vi "set_mirrors_from_EoF.vi"(1 "offset Y":dbl, 3 "offset X":dbl, 4 "Line_start":i32, 5 "Range":dbl=10.0, 6 "Pixels":i32=256, 7 "dwell":dbl=1.0) -> (0 "X and Y":waveform(dbl)[](array[waveform]), 2 "appended array":dbl[][](array[numeric]))   [LabVIEW 2016]
panel:
  out "start frame Y Volts 2":dbl
  out "Waveform Graph 2":dbl[](graph)
  out "start frame Y Volts":dbl
  out "Waveform Graph":waveform(dbl)[](graph)
  out "border of frame X Volts":dbl
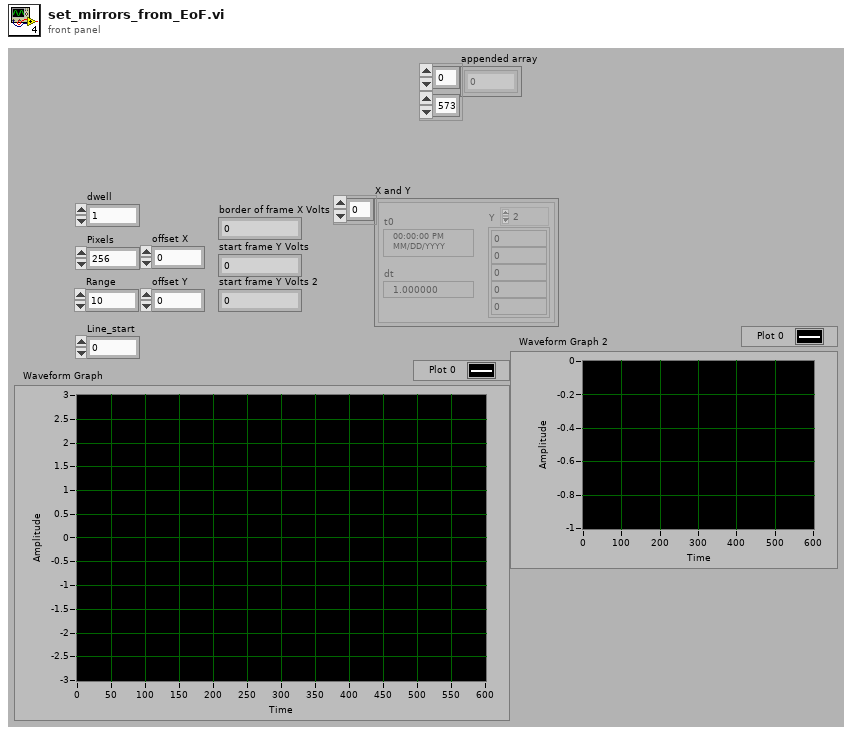
[diagram p1: front panel]
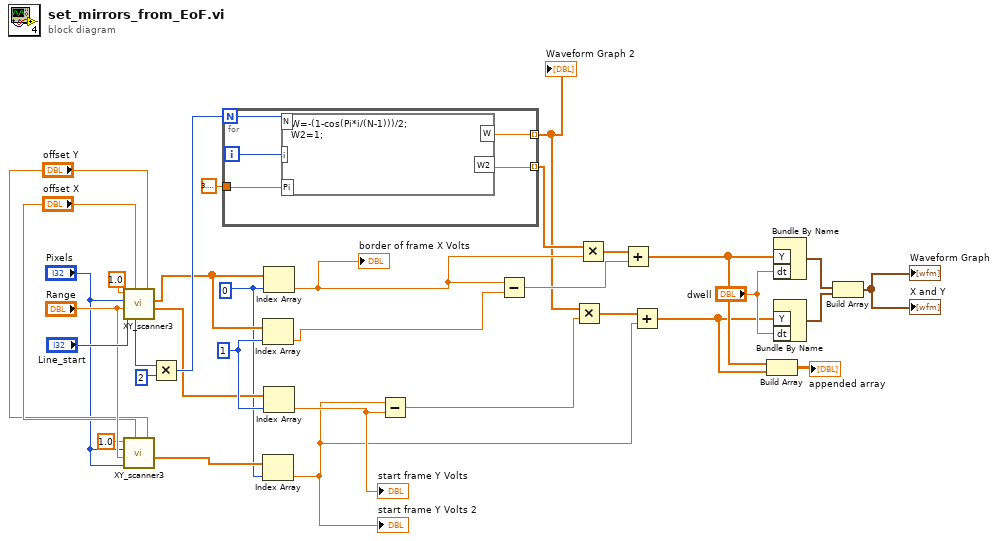
[diagram p0: block diagram]
diagram:
  w1 = 0 ("index")
  w3 = 1 ("index")
  n1 = call "XY_scanner3.vi"("offset Y"="offset Y", "offset X"="offset X", "Line_start"="Line_start", "Range"="Range", "Pixels"="Pixels", "dwell"=1.0) -> ("Array Y"=w2:dbl[], "Array X"=w4:dbl[], "scanPix"=w15:i32)  [unwired: 1 out]
  n2 = call "XY_scanner3.vi"("offset Y"="offset Y", "offset X"="offset X", "Line_start"="Pixels", "Range"="Range", "Pixels"="Pixels", "dwell"=1.0) -> ("Array Y"=w14:dbl[])  [unwired: 3 out]
  n3 = Multiply(x=w15, y=2) -> (x*y=w20:i32)
  n4 = for {
    N: w20 -> [w37]
    tunnel: 3.141592653589793 -> [w36]
    tunnel: [w35] -> w7 mode=indexing
    tunnel: [w34] -> w25 mode=indexing
    i -> [w38]
    n5 = formula code="W=-(1-cos(Pi*i/(N-1)))/2;\nW2=1;"("N"=w37, "i"=w38, "Pi"=w36) -> ("W"=w35:dbl, "W2"=w34:dbl)
  }
  "Waveform Graph 2" <- w7
  n6 = Index Array(array=w4, index=w3) -> (element=w12:dbl)
  n7 = Index Array(array=w14, index=w1) -> (element=w5:dbl)
  "start frame Y Volts 2" <- w5
  n8 = Index Array(array=w4, index=w1) -> (element=w11:dbl)
  "border of frame X Volts" <- w11
  n9 = Index Array(array=w2, index=w3) -> (element=w6:dbl)
  "start frame Y Volts" <- w6
  n10 = Subtract(x=w5, y=w6) -> (x-y=w8:dbl)
  n11 = Subtract(x=w11, y=w12) -> (x-y=w24:dbl)
  n12 = Multiply(x=w7, y=w8) -> (x*y=w10:dbl[])
  n13 = Multiply(x=w25, y=w11) -> (x*y=w23:dbl[])
  n14 = Add(x=w23, y=w24) -> (x+y=w22:dbl[])
  n15 = Add(x=w10, y=w5) -> (x+y=w9:dbl[])
  n16 = Build Array(w22, w9) -> (→"appended array":dbl[][])
  n17 = Bundle By Name("Y"=w22, "dt"="dwell") -> (w31:waveform(dbl))  [unwired: 1 in]
  n18 = Bundle By Name("Y"=w9, "dt"="dwell") -> (w30:waveform(dbl))  [unwired: 1 in]
  n19 = Build Array(w31, w30) -> (→"X and Y" →"Waveform Graph":waveform(dbl)[])
